vi "delete_element(variant).vi"(8 "error in (no error)":errorcluster, 10 "name":string, 11 "data store (in)":variant) -> (0 "error out":errorcluster, 2 "found":bool, 3 "data store (out)":variant)   [LabVIEW 2018]
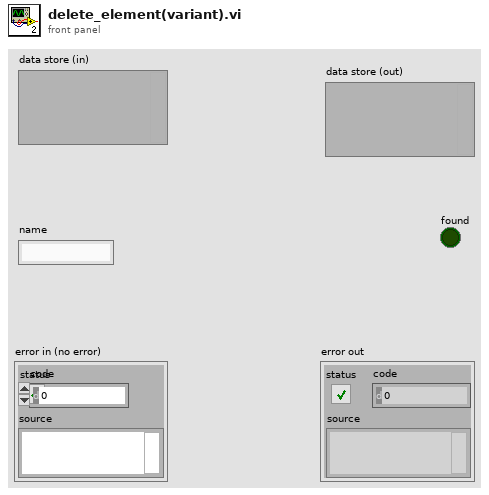
[diagram p1: front panel]
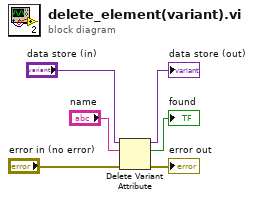
[diagram p0: block diagram]
diagram:
  n1 = Delete Variant Attribute(4:"error in (no error)", 6:"name", 7:"data store (in)") -> (0:→"error out":errorcluster, 2:→"found":bool, 3:→"data store (out)":variant)
